vi "Q_Split.vi"(8 "error in":errorcluster caption="错误输入（无错误）", 10 "Split Mode":T1, 11 "ChildNode*":refnum<data-value>) -> (0 "error out":errorcluster caption="错误输出")   [LabVIEW 2013, in "PanelDataNode.lvclass"]
uses:
  PanelDataNode.lvclass
  Split Mode.ctl
  PanelDataNode.lvclass/PanelDataNode.ctl
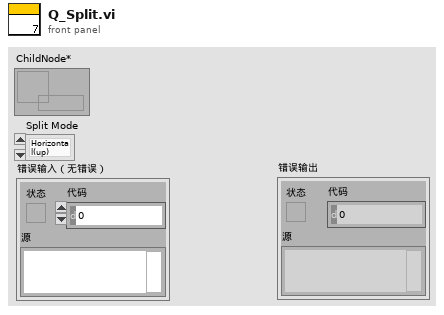
[diagram p1: front panel]
types:
  T1 = typedef "PanelDataNode.lvclass/Split Mode.ctl" = enum16{"Horizontal(up)", "Vertical(left)", "Horizontal(down)", "Vertical(right)"}
  T2 = cluster{"ChildNode*":refnum<data-value>, "Split Mode":T1}
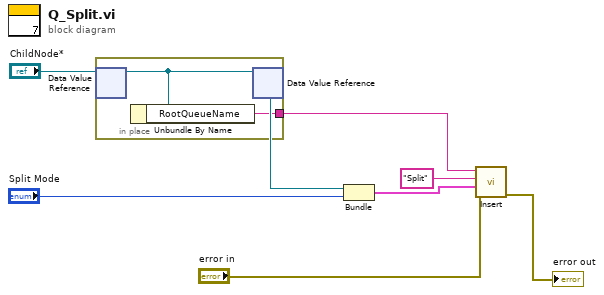
[diagram p0: block diagram]
diagram:
  n1 = in-place {
    in-place-border: [w9] -> w3
    n2 = in-place-dvr #1("ChildNode*") -> (w10:refnum<class "PanelDataNode.lvclass">)  [unwired: 1 out]
    n3 = Unbundle By Name(w10) -> ("RootQueueName"=w9:string)
    n4 = in-place-dvr #1(w10) -> (w4:refnum<data-value>)  [unwired: 1 out]
  }
  n5 = Bundle("ChildNode*"=w4, "Split Mode"="Split Mode") -> (w7:T2)  [unwired: 1 in]
  n6 = call "Insert.vi"("error in"="error in", "Data"=w7, "Event"="Split", "QueueName"=w3) -> ("error out"=→"error out":errorcluster)  [unwired: 6 in, 1 out]
